vi "cRIO Main.vi"() -> ()   [LabVIEW 2013]
uses:
  Engine Command Receiver/SubVIs/command commands to rtexe process.ctl
  Engine Command Receiver/SubVIs/engine status data.ctl
  <vilib>/NI/Module Execution Interface/Engine Runtime/Execution States.ctl
  Engine Command Receiver/SubVIs/queue name.ctl
  <vilib>/NI/Current Value Table/DataTypes/Double_Read.vi
  <vilib>/NI/Current Value Table/DataTypes/Boolean_Write.vi
  <vilib>/NI/Current Value Table/DataTypes/Double_Write.vi
  <vilib>/NI/Current Value Table/Type to Enum.vi
  <vilib>/NI/Current Value Table/DataTypes/Double_Type To Enum.vi
  <vilib>/NI/Current Value Table/DataTypes/Boolean_Type To Enum.vi
  <vilib>/NI/AMC/Read Termination Message.vi
  Engine Command Receiver/SubVIs/command to string.vi
  Engine Command Receiver/SubVIs/string to commands.vi
  <vilib>/NI/AMC/Create Single Message.vi
  <vilib>/NI/Current Value Table/FGVs/CVT Globals.vi
  <vilib>/NI/Current Value Table/FGVs/Tag Memory.vi
  <vilib>/NI/Current Value Table/Memory Block.vi
  <vilib>/NI/Current Value Table/DataTypes/Boolean_Memory Block.vi
  <vilib>/NI/Current Value Table/DataTypes/Double_Memory Block.vi
  <vilib>/NI/AMC/Globals.vi
  Engine Command Receiver/module execution process.lvlib
  <vilib>/NI/AMC/AMC.lvlib
  <vilib>/NI/Current Value Table/Current Value Table.lvlib
  <vilib>/NI/Module Execution Interface/Engine Runtime/Engine Runtime Interface.lvclass
panel:
  in  "Pause":bool
  out "Scan Engine Period":u32
  in  "Exit":bool
  in  "Reload":bool
  out "timed structures load":dbl
  out "CPU load average":dbl
  out "error out":errorcluster
  out "Lamp PWM":cluster{"Value":dbl, "Value":dbl}(graph)
  out "Temperature":cluster{"Value":dbl, "Value":dbl}(graph)
  in  "Fan on?":bool
  in  "Setpoint":dbl=25.0
  out "system error":errorcluster
  out "engine statuses":T1[](array[typedef])
  out "command error":errorcluster
  out "commands":T3
  out "engine loaded":string
  out "load error":errorcluster
  out "Invalid Message":string
  in  "config. file path":path=path "/home/lvuser/natinst/bin/SimulatedSystem.pcfg"
  # "Status Information"
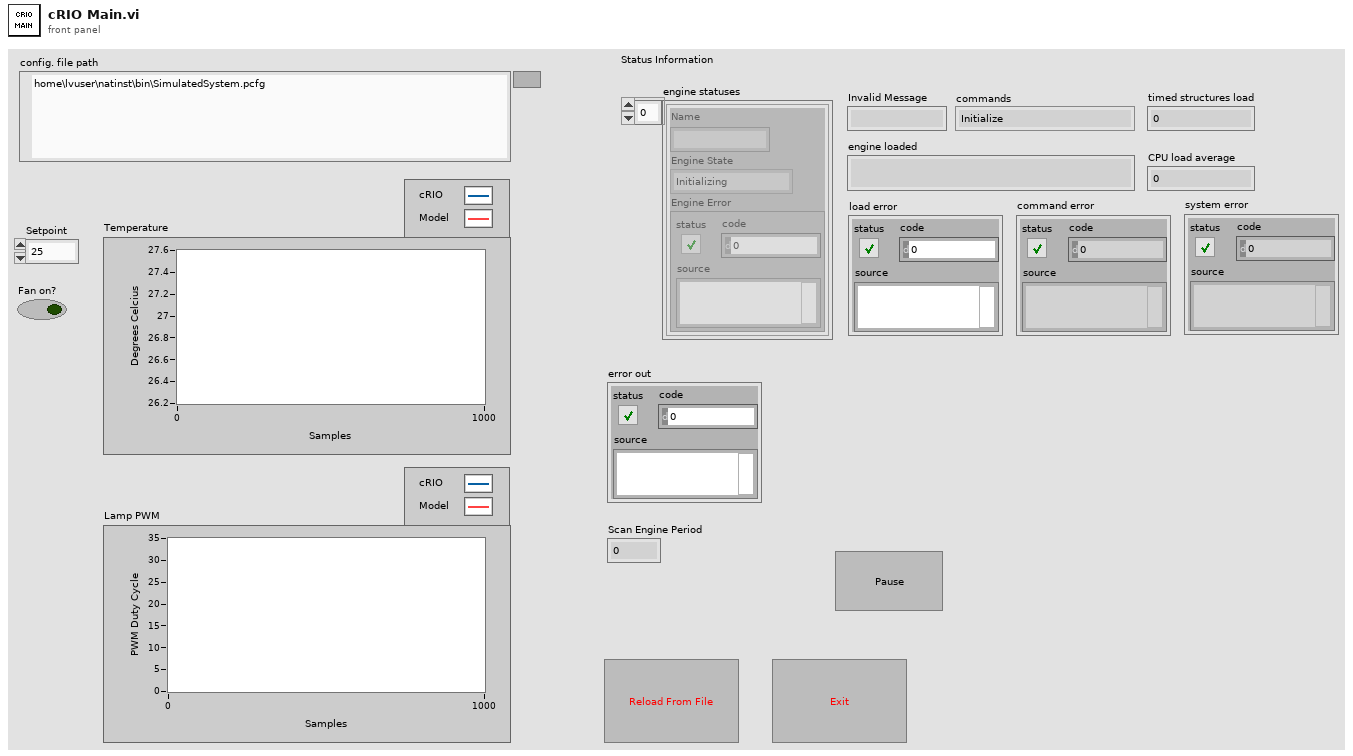
[diagram p1: front panel]
types:
  T1 = typedef "module execution process.lvlib/engine status data.ctl" = cluster{"Name":string, "Engine State":T2, "Engine Error":errorcluster}
  T2 = typedef "Engine Runtime Interface.lvclass/Execution States.ctl" = enum16{"Initializing", "Paused (Initialized)", "Running", "Set Safe Outputs", "Uninitializing", "Stopped (Uninitialized)", "Error (Uninitialized)", "Safe State (Uninitialized)", "Closed"}
  T3 = typedef "module execution process.lvlib/command commands to rtexe process.ctl" = enum16{"Initialize", "Load from File", "Load from String", "Open All Engines", "Open Single Engine", "Initialize All Engines", "Initialize Single Engine", "Start All", "Start Single", "Pause All", "Pause Single", "Stop All", "Stop Single", "Close All", "Close Single", "Set Safe State All", "Set Safe State Single", "Get Status", "Exit", "Error", "Load Bitfile", "Unload Bitfile", "Add Search Paths"}
  T4 = typedef "module execution process.lvlib/queue name.ctl" = enum16{"TOrtmainexec", "FROMrtmainexec"}
  T5 = typedef "AMC.lvlib/Message Queue.ctl" = refnum<queue>
  T6 = typedef "module execution process.lvlib/common reponses to network process.ctl" = enum16{"System Error", "Load Report", "Action Response", "Engine Status"}
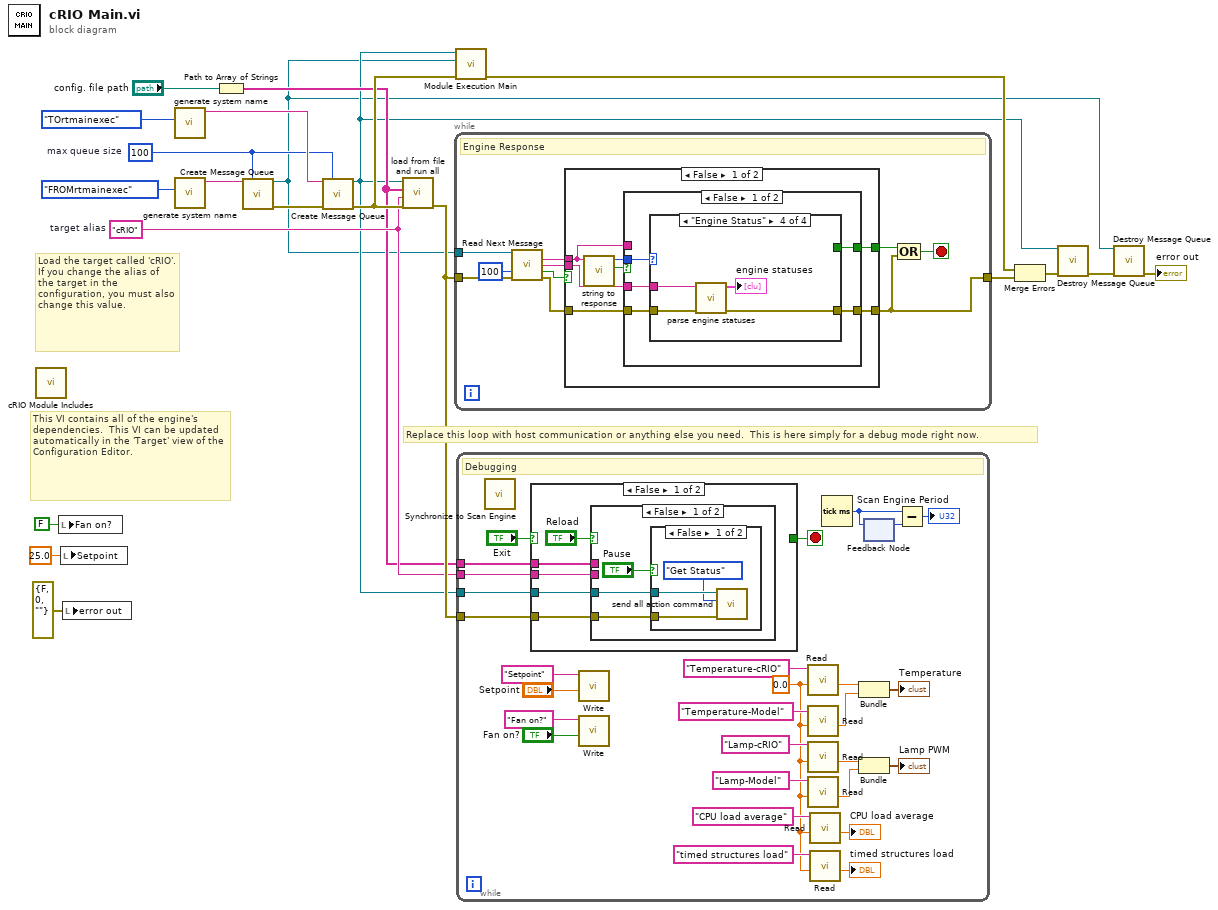
[diagram p0: block diagram]
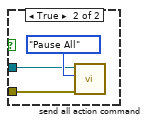
[diagram p2: hidden frame]
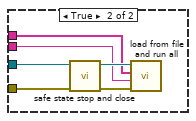
[diagram p3: hidden frame]
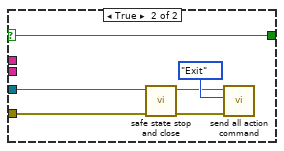
[diagram p4: hidden frame]
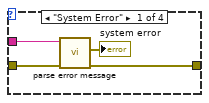
[diagram p5: hidden frame]
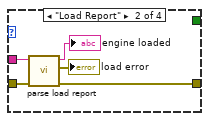
[diagram p6: hidden frame]
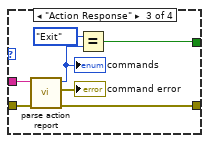
[diagram p7: hidden frame]
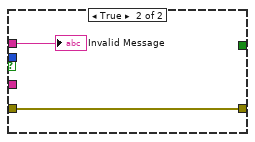
[diagram p8: hidden frame]
diagram:
  w15 = 100  # max queue size
  w9 = "cRIO"  # target alias
  # "This VI contains all of the engine's dependencies.  This VI can be updated automatically in the 'Target' view of the Configuration Editor."
  # "Load the target called 'cRIO'.  If you change the alias of the target in the configuration, you must also change this value."
  # "Replace this loop with host communication or anything else you need.  This is here simply for a debug mode right now."
  n1 = call "cRIO Module Includes.vi"() -> ()  [unwired: 12 in]
  n2 = local write "Fan on?"(FALSE ("Fan on?")) -> ()
  n3 = local write "Setpoint"(25.0 ("Setpoint")) -> ()
  n4 = local write "error out"(errorcluster {"status"=FALSE, "code"=0, "source"=""} ("error out")) -> ()
  n5 = call "generate system name.vi"("queue"=queue_name."TOrtmainexec") -> ("queue name"=w19:string)  [unwired: 10 in]
  n6 = call "generate system name.vi"("queue"=queue_name."FROMrtmainexec") -> ("queue name"=w21:string)  [unwired: 10 in]
  n7 = Path to Array of Strings(0:"config. file path") -> (2:w8:string[])  [unwired: 1 out]
  n8 = call <vilib>:"Create Message Queue.vi"("message queue name"=w21, "max queue size (-1, unlimited)"=w15) -> ("message queue out"=w1:T5, "error out"=w20:errorcluster)  [unwired: 12 in]
  n9 = call <vilib>:"Create Message Queue.vi"("message queue name"=w19, "max queue size (-1, unlimited)"=w15, "error in"=w20) -> ("message queue out"=w2:T5, "error out"=w11:errorcluster)  [unwired: 11 in]
  n10 = call "load from file and run all.vi"("error in"=w11, "target alias"=w9, "tokenized path"=w8, "message queue in"=w2) -> ("error out"=w10:errorcluster)  [unwired: 6 in, 1 out]
  n11 = while {
    tunnel: w1 -> [w30]
    tunnel: w10 -> [w27]
    tunnel: [w22] -> w7
    stop <- w24 stop-if-true
    # "Engine Response"
    n12 = call <vilib>:"Read Next Message.vi"("message queue in"=w30, "timeout (1 ms)"=100, "error in"=w27) -> ("message name"=w29:string, "message value"=w23:string, "timed out?"=w26:bool, "error out"=w28:errorcluster)  [unwired: 5 in, 4 out]
    n13 = case shown="False" w26 {
      tunnel: w29 -> [w32 _]
      tunnel: [w37 _] -> w25
      tunnel: w28 -> [w35 w66]
      tunnel: [w34 w66] -> w22
      tunnel: w23 -> [w33 _]
      frame False {
        n14 = call "string to response.vi"("command string"=w32) -> ("invalid"=w38:bool, "responses"=w36:T6)  [unwired: 9 in]
        n15 = case shown="False" w38 {
          tunnel: w33 -> [w42 _]
          tunnel: [w39 _] -> w37
          tunnel: w36 -> [w43 _]
          tunnel: w35 -> [w41 w65]
          tunnel: [w40 w65] -> w34
          tunnel: w32 -> [_ w64]
          frame False {
            n16 = case shown="\"Engine Status\"" w43 {
              tunnel: w42 -> [w47 w52 w59 w63]
              tunnel: w41 -> [w46 w51 w58 w62]
              tunnel: [w44 w48 w56 w61] -> w40
              tunnel: [_ _ w53 _] -> w39
              frame "System Error" {
                n17 = call "parse error message.vi"("error in"=w46, "message data"=w47) -> ("error out"=w44:errorcluster, "system error"=→"system error":errorcluster)  [unwired: 8 in]
              }
              frame "Load Report" {
                n18 = call "parse load report.vi"("error in"=w51, "message data"=w52) -> ("error out"=w48:errorcluster, "load error"=→"load error":errorcluster, "engine loaded"=→"engine loaded":string)  [unwired: 7 in]
              }
              frame "Action Response" {
                n19 = call "parse action report.vi"("error in"=w58, "message data"=w59) -> ("error out"=w56:errorcluster, "command error"=→"command error":errorcluster, "commands"=w55:T3)  [unwired: 7 in]
                "commands" <- w55
                n20 = Equal?(x=command_commands_to_rtexe_process."Exit", y=w55) -> (x = y?=w53:bool)
              }
              frame "Engine Status" {
                n21 = call "parse engine statuses.vi"("error in"=w62, "message data"=w63) -> ("error out"=w61:errorcluster, "engine statuses"=→"engine statuses":T1[])  [unwired: 8 in]
              }
            }
          }
          frame True {
            "Invalid Message" <- w64
          }
        }
      }
      frame True {
      }
    }
    n22 = Compound Arithmetic op=OR(w25, w22) -> (w24:bool)
  }
  n23 = call "Module Execution Main.vi"("error in"=w11, "response queue"=w1, "command queue"=w2) -> ("error out"=w6:errorcluster)  [unwired: 8 in]
  n24 = while {
    tunnel: w10 -> [w73]
    tunnel: w2 -> [w74]
    tunnel: w8 -> [w72]
    tunnel: w9 -> [w71]
    stop <- w67 stop-if-true
    w78 = 0.0 ("Default")
    # "Debugging"
    n25 = call <vilib>:"Synchronize to Scan Engine.vi"() -> ()  [unwired: 10 in, 2 out]
    n26 = case shown="False" "Exit" {
      selector: "Exit" -> [_ w118]
      tunnel: w74 -> [w98 w120]
      tunnel: w73 -> [w97 w119]
      tunnel: w72 -> [w96 _]
      tunnel: w71 -> [w95 _]
      tunnel: [_ w118] -> w67
      frame False {
        n27 = case shown="False" "Reload" {
          tunnel: w98 -> [w102 w114]
          tunnel: w97 -> [w101 w113]
          tunnel: w96 -> [_ w110]
          tunnel: w95 -> [_ w109]
          frame False {
            n28 = case shown="False" "Pause" {
              tunnel: w102 -> [w105 w107]
              tunnel: w101 -> [w104 w106]
              frame False {
                n29 = call "send all action command.vi"("error in"=w104, "commands"=command_commands_to_rtexe_process."Get Status", "message queue in"=w105) -> ()  [unwired: 7 in, 2 out]
              }
              frame True {
                n30 = call "send all action command.vi"("error in"=w106, "commands"=command_commands_to_rtexe_process."Pause All", "message queue in"=w107) -> ()  [unwired: 7 in, 2 out]
              }
            }
          }
          frame True {
            n31 = call "safe state stop and close.vi"("error in"=w113, "message queue in"=w114) -> ("error out"=w111:errorcluster, "message queue out"=w112:T5)  [unwired: 8 in]
            n32 = call "load from file and run all.vi"("error in"=w111, "target alias"=w109, "tokenized path"=w110, "message queue in"=w112) -> ()  [unwired: 6 in, 2 out]
          }
        }
      }
      frame True {
        n33 = call "safe state stop and close.vi"("error in"=w119, "message queue in"=w120) -> ("error out"=w115:errorcluster, "message queue out"=w116:T5)  [unwired: 8 in]
        n34 = call "send all action command.vi"("error in"=w115, "commands"=command_commands_to_rtexe_process."Exit", "message queue in"=w116) -> ()  [unwired: 7 in, 2 out]
      }
    }
    n35 = call-poly <vilib>:"Write.vi"("Value"="Setpoint", "Tag Name"="Setpoint") -> ()  [unwired: 9 in, 1 out]
    n36 = call-poly <vilib>:"Write.vi"("Value"="Fan on?", "Tag Name"="Fan on?") -> ()  [unwired: 9 in, 1 out]
    n37 = call-poly <vilib>:"Read.vi"("Default"=w78, "Tag Name"="Temperature-cRIO") -> ("Value"=w86:dbl)  [unwired: 8 in, 1 out]
    n38 = call-poly <vilib>:"Read.vi"("Default"=w78, "Tag Name"="Temperature-Model") -> ("Value"=w85:dbl)  [unwired: 8 in, 1 out]
    n39 = call-poly <vilib>:"Read.vi"("Default"=w78, "Tag Name"="Lamp-cRIO") -> ("Value"=w84:dbl)  [unwired: 8 in, 1 out]
    n40 = call-poly <vilib>:"Read.vi"("Default"=w78, "Tag Name"="Lamp-Model") -> ("Value"=w83:dbl)  [unwired: 8 in, 1 out]
    n41 = call-poly <vilib>:"Read.vi"("Default"=w78, "Tag Name"="CPU load average") -> ("Value"=→"CPU load average":dbl)  [unwired: 8 in, 1 out]
    n42 = call-poly <vilib>:"Read.vi"("Default"=w78, "Tag Name"="timed structures load") -> ("Value"=→"timed structures load":dbl)  [unwired: 8 in, 1 out]
    n43 = Tick Count (ms)() -> (millisecond timer value=w69:u32)
    n44 = Bundle("Value"=w86, "Value"=w85) -> (→"Temperature":cluster{"Value":dbl, "Value":dbl})  [unwired: 1 in]
    n45 = Bundle("Value"=w84, "Value"=w83) -> (→"Lamp PWM":cluster{"Value":dbl, "Value":dbl})  [unwired: 1 in]
    n46 = feedback-in #1(w69) -> ()
    n47 = feedback #1() -> (w70:u32)  [unwired: 1 in]
    n48 = Subtract(x=w69, y=w70) -> (x-y=→"Scan Engine Period":u32)
  }
  n49 = Merge Errors(w6, w7) -> (w3:errorcluster)
  n50 = call <vilib>:"Destroy Message Queue.vi"("message queue in"=w2, "error in"=w3) -> ("error out"=w5:errorcluster)  [unwired: 11 in, 2 out]
  n51 = call <vilib>:"Destroy Message Queue.vi"("message queue in"=w1, "error in"=w5) -> ("error out"=→"error out":errorcluster)  [unwired: 11 in, 2 out]
